vi "!_Serial_log_builder.vi"(0 "Port Name":string, 1 "Comms Error":bool, 2 "Channel Name":string, 3 "Write String":string, 4 "Log Errors?":bool, 5 "Read":string) -> ()   [LabVIEW 2022 SP3]
uses:
  ADAM Client/Sub VIs/ADAM Controls/Remember_value_mode.ctl
  Serial_Logging_Global.vi
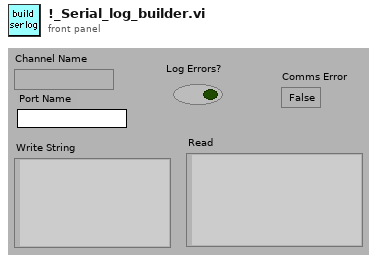
[diagram p1: front panel]
types:
  T1 = typedef "Remember_value_mode.ctl" = enum16{"Read only", "Read and Write"}
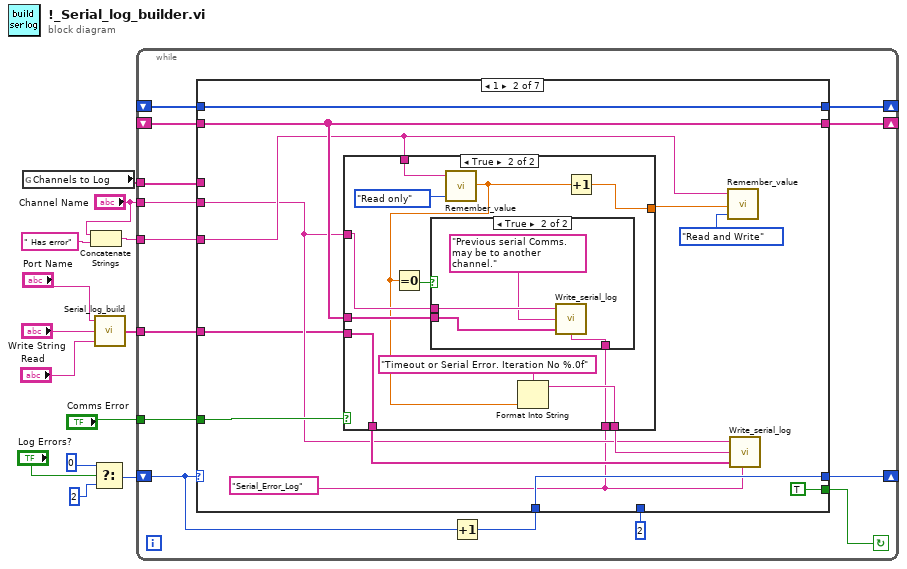
[diagram p0: block diagram]
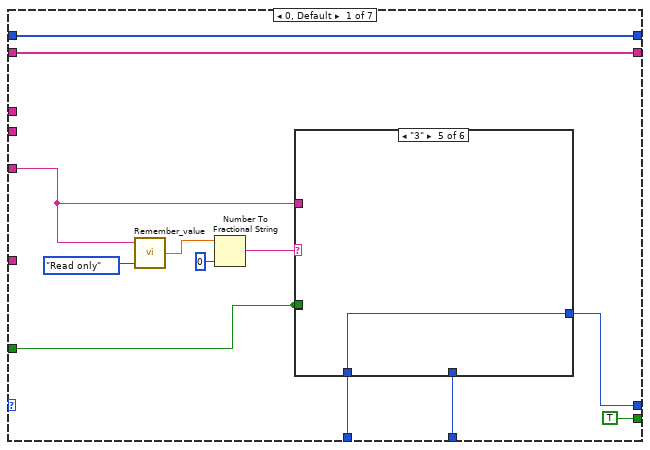
[diagram p2: hidden frame]
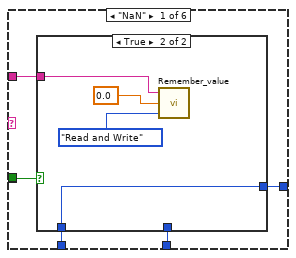
[diagram p3: hidden frame]
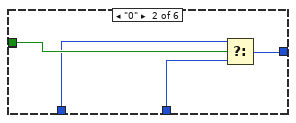
[diagram p5: hidden frame]
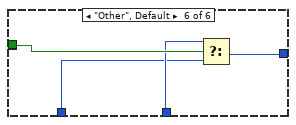
[diagram p8: hidden frame]
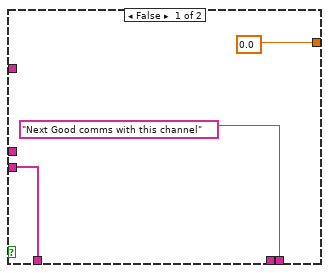
[diagram p9: hidden frame]
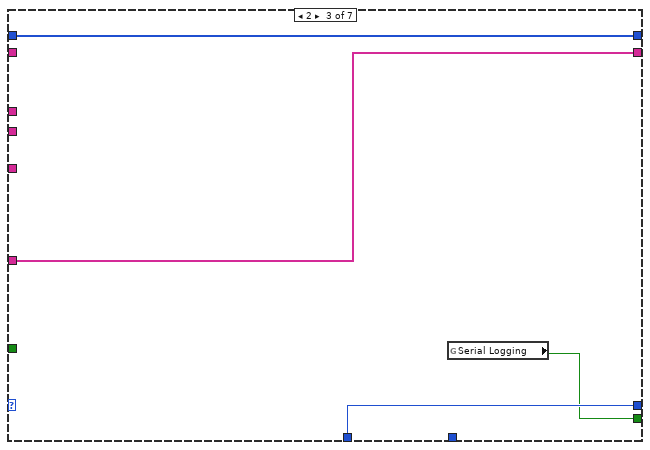
[diagram p11: hidden frame]
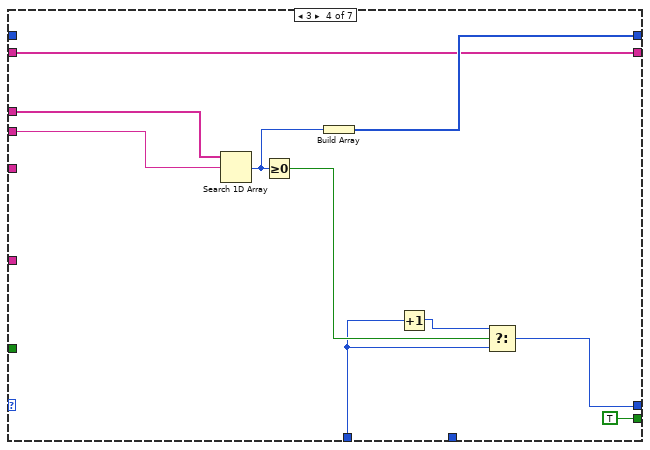
[diagram p12: hidden frame]
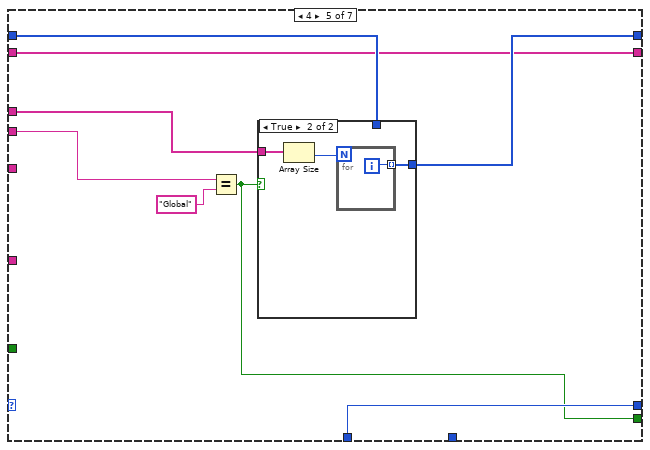
[diagram p13: hidden frame]
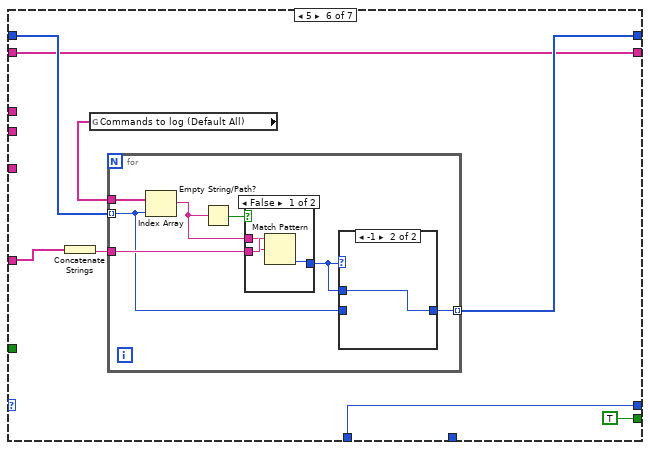
[diagram p15: hidden frame]
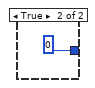
[diagram p16: hidden frame]
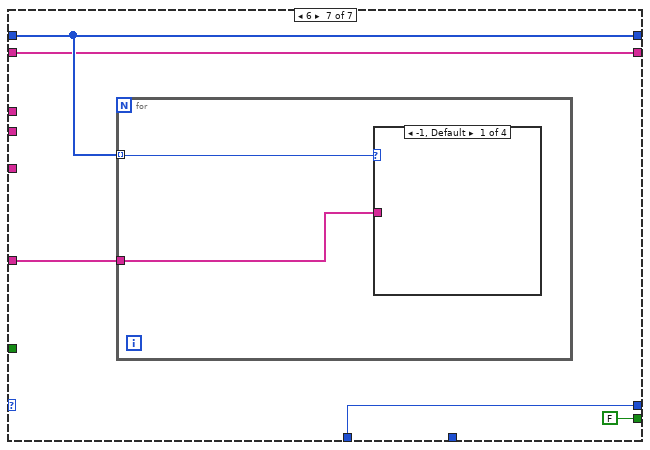
[diagram p18: hidden frame]
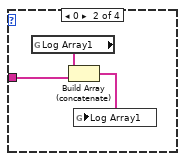
[diagram p19: hidden frame]
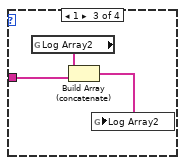
[diagram p20: hidden frame]
diagram:
  n1 = global read "Serial_Logging_Global.vi" "Channels to Log"() -> (w13:string[])
  n2 = Concatenate Strings("Channel Name", " Has error" ("Substring")) -> (w10:string)
  n3 = Select(t=0, s="Log Errors?", f=2) -> (s? t:f=w1:i32)
  n4 = call "Serial_log_build.vi"("Read"="Read", "Write String"="Write String", "Port Name"="Port Name") -> ("Output Array"=w5:string[])
  n5 = while {
    tunnel: w5 -> [w14]
    tunnel: "Comms Error" -> [w16]
    tunnel: w10 -> [w17]
    shift-left: _ -> [w18]
    shift-right: [w19] -> _
    shift-left: _ -> [w20]
    shift-right: [w21] -> _
    tunnel: "Channel Name" -> [w22]
    tunnel: w13 -> [w23]
    shift-left: w1 -> [w26]
    shift-right: [w24] -> _
    stop <- w27 continue-if-true
    n6 = Increment(x=w26) -> (x+1=w25:i32)
    n7 = case shown="1" w26 {
      tunnel: [TRUE ("Serial Logging") TRUE ("Serial Logging") w94 TRUE ("Serial Logging") w108 TRUE ("Serial Logging") FALSE ("Serial Logging")] -> w27
      tunnel: w25 -> [w31 w72 w95 w98 w113 w126 w144]
      tunnel: [w32 w72 w95 w97 w113 w126 w144] -> w24
      tunnel: w23 -> [_ _ _ w105 w110 _ _]
      tunnel: w22 -> [_ w63 _ w104 w109 _ _]
      tunnel: [w39 w73 w93 w102 w111 w122 w143] -> w21
      tunnel: w20 -> [w39 w73 w93 _ w107 w124 w143]
      tunnel: [w37 w66 w92 w96 w106 w120 w141] -> w19
      tunnel: w18 -> [w37 w66 _ w96 w106 w120 w141]
      tunnel: w17 -> [w33 w64 _ _ _ _ _]
      tunnel: w16 -> [w29 w67 _ _ _ _ _]
      tunnel: 2 -> [w30 _ _ _ _ _ _]
      tunnel: w14 -> [_ w62 w92 _ _ w119 w140]
      frame 0, Default {
        n8 = call "Remember_value.vi"("Mode"=Remember_value_mode."Read only", "Ch name"=w33) -> ("Output Value"=w35:dbl)  [unwired: 1 in]
        n9 = Number To Fractional String(number=w35, precision (6)=i16 0) -> (F-format string=w34:string)  [unwired: 2 out]
        n10 = case shown="\"3\"" w34 {
          tunnel: w29 -> [w44 _ _ _ _ w60]
          tunnel: w33 -> [w43 _ _ _ _ _]
          tunnel: [w41 w50 w54 w55 w56 w57] -> w32
          tunnel: w31 -> [w42 w52 w54 w55 w56 w58]
          tunnel: w30 -> [w40 w51 _ _ _ w59]
          tunnel: w29 -> [_ w53 _ _ _ _]
          frame "NaN" {
            n11 = case shown="True" w44 {
              tunnel: w43 -> [_ w47]
              tunnel: w42 -> [_ w46]
              tunnel: [w45 w46] -> w41
              tunnel: w40 -> [w45 _]
              frame False {
              }
              frame True {
                n12 = call "Remember_value.vi"("Mode"=Remember_value_mode."Read and Write", "Input Value"=0.0, "Ch name"=w47) -> ()  [unwired: 1 out]
              }
            }
          }
          frame "0" {
            n13 = Select(t=w52, s=w53, f=w51) -> (s? t:f=w50:i32)
          }
          frame "1" {
          }
          frame "2" {
          }
          frame "3" {
          }
          frame "Other", Default {
            n14 = Select(t=w59, s=w60, f=w58) -> (s? t:f=w57:i32)
          }
        }
      }
      frame 1 {
        w61 = "Serial_Error_Log" ("Log Type")
        n15 = case shown="True" w67 {
          tunnel: ["Next Good comms with this channel" ("Header message") w78] -> w68
          tunnel: [0.0 ("Input Value") w85] -> w69
          tunnel: w66 -> [_ w81]
          tunnel: w62 -> [w74 w84]
          tunnel: [w74 w84] -> w65
          tunnel: w64 -> [_ w86]
          tunnel: w63 -> [_ w82]
          tunnel: w61 -> [_ w77]
          frame False {
          }
          frame True {
            n16 = call "Remember_value.vi"("Mode"=Remember_value_mode."Read only", "Ch name"=w86) -> ("Output Value"=w80:dbl)  [unwired: 1 in]
            n17 = Equal To 0?(x=w80) -> (x = 0?=w83:bool)
            n18 = case shown="True" w83 {
              tunnel: w82 -> [_ w91]
              tunnel: w81 -> [_ w89]
              tunnel: w77 -> [_ w88]
              frame False {
              }
              frame True {
                n19 = call "Write_serial_log.vi"("Log Type"=w88, "Log Array"=w89, "Header message"="Previous serial Comms. may be to another channel.", "Channel Name"=w91) -> ()  [unwired: 1 out]
              }
            }
            n20 = Format Into String(format string="Timeout or Serial Error. Iteration No %.0f" ("Format String"), w80) -> (resulting string=w78:string)  [unwired: 2 in, 1 out]
            n21 = Increment(x=w80) -> (x+1=w85:dbl)
          }
        }
        n22 = call "Remember_value.vi"("Mode"=Remember_value_mode."Read and Write", "Input Value"=w69, "Ch name"=w64) -> ()  [unwired: 1 out]
        n23 = call "Write_serial_log.vi"("Log Type"=w61, "Log Array"=w65, "Header message"=w68, "Channel Name"=w63) -> ()  [unwired: 1 out]
      }
      frame 2 {
        n24 = global read "Serial_Logging_Global.vi" "Serial Logging"() -> (w94:bool)
      }
      frame 3 {
        n25 = Search 1D Array(1D array=w105, element=w104) -> (index of element=w103:i32)  [unwired: 1 out]
        n26 = Greater Or Equal To 0?(x=w103) -> (x >= 0?=w100:bool)
        n27 = Build Array(w103) -> (w102:i32[])
        n28 = Increment(x=w98) -> (x+1=w99:i32)
        n29 = Select(t=w99, s=w100, f=w98) -> (s? t:f=w97:i32)
      }
      frame 4 {
        n30 = Equal?(x=w109, y="Global") -> (x = y?=w108:bool)
        n31 = case shown="True" w108 {
          tunnel: w110 -> [_ w117]
          tunnel: [w114 w115] -> w111
          tunnel: w107 -> [w114 _]
          frame False {
          }
          frame True {
            n32 = Array Size(array=w117) -> (size(s)=w116:i32)
            n33 = for {
              N: w116 -> [_]
              tunnel: [w118] -> w115 mode=indexing
              i -> [w118]
            }
          }
        }
      }
      frame 5 {
        n34 = Concatenate Strings(w119) -> (w125:string)
        n35 = global read "Serial_Logging_Global.vi" "Commands to log (Default All)"() -> (w123:string[])
        n36 = for {
          tunnel: w125 -> [w133]
          tunnel: w124 -> [w130] mode=indexing
          tunnel: w123 -> [w132]
          tunnel: [w131] -> w122 mode=indexing
          n37 = Index Array(array=w132, index=w130) -> (element=w129:string)
          n38 = Empty String/Path?(string/path=w129) -> (empty?=w128:bool)
          n39 = case shown="False" w128 {
            tunnel: w133 -> [w136 _]
            tunnel: w129 -> [w135 _]
            tunnel: [w134 0 ("offset past match")] -> w127
            frame False {
              n40 = Match Pattern(string=w136, regular expression=w135) -> (offset past match=w134:i32)  [unwired: 4 out]
            }
            frame True {
            }
          }
          n41 = case shown="-1" w127 {
            tunnel: [w138 w139] -> w131
            tunnel: w130 -> [w138 _]
            tunnel: w127 -> [_ w139]
            frame 0, Default {
            }
            frame -1 {
            }
          }
        }
      }
      frame 6 {
        n42 = for {
          tunnel: w143 -> [w146] mode=indexing
          tunnel: w140 -> [w145]
          n43 = case shown="-1, Default" w146 {
            tunnel: w145 -> [_ w147 w150 w153]
            frame -1, Default {
            }
            frame 0 {
              n44 = global read "Serial_Logging_Global.vi" "Log Array1"() -> (w149:string[])
              n45 = Build Array (concatenate)(w149, w147) -> (w148:string[])
              n46 = global write "Serial_Logging_Global.vi" "Log Array1"(w148) -> ()
            }
            frame 1 {
              n47 = global read "Serial_Logging_Global.vi" "Log Array2"() -> (w152:string[])
              n48 = Build Array (concatenate)(w152, w150) -> (w151:string[])
              n49 = global write "Serial_Logging_Global.vi" "Log Array2"(w151) -> ()
            }
            frame 2 {
              n50 = global read "Serial_Logging_Global.vi" "Log Array3"() -> (w155:string[])
              n51 = Build Array (concatenate)(w155, w153) -> (w154:string[])
              n52 = global write "Serial_Logging_Global.vi" "Log Array3"(w154) -> ()
            }
          }
        }
      }
    }
  }
